vi "AddOption_Axes.vi"(0 "reference in":refnum<class "HTMLPlot.lvclass">, 2 "OptionsIn":string[](array[string]), 5 "error in (no error)":errorcluster) -> (14 "reference out":refnum<class "HTMLPlot.lvclass">, 16 "OptionsOut":string[](array[string]), 19 "error out":errorcluster)   [LabVIEW 2019, in "HTMLPlot.lvclass"]
uses:
  HTMLPlot.lvclass
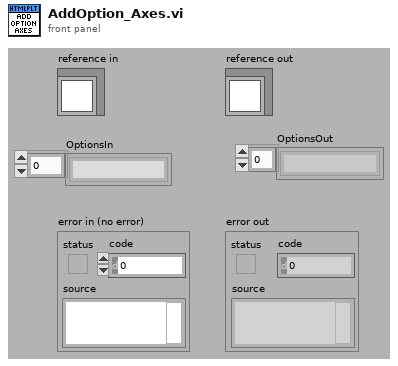
[diagram p1: front panel]
types:
  T1 = typedef "HTMLPlot.lvclass/ObjectAttributes.ctl" = cluster{"Attribute1":dbl, "GraphContainer":refnum<k7>, "ChartScriptFile":string, "UtilScriptFile(demoData)":string, "BaseHTML":string, "GenericProperties":cluster{"PlotType":T2, "PlotTitle":string, "XLabel":string, "YLabel":string, "ShowToolTip":bool}, "LegendProperties":cluster{"Show":bool, "Position":T3}, "BarPlot":cluster{"Dataset":dbl[][], "DatasetLabels":string[], "XLabels":string[], "PlotColours":u32[], "Stacked":bool}, "PiePlot":cluster{"Dataset":dbl[][], "DatasetLabels":string[], "PlotColours":u32[], "DoughnutStyle":bool, "PlotLabels":string[]}, "connection ID":refnum<k5>, "PortID":u64}
  T2 = typedef "HTMLPlot.lvclass/PlotType.ctl" = enum16{"bar", "line", "pie"}
  T3 = typedef "HTMLPlot.lvclass/LegendPosition.ctl" = enum16{"top", "right", "left", "bottom"}
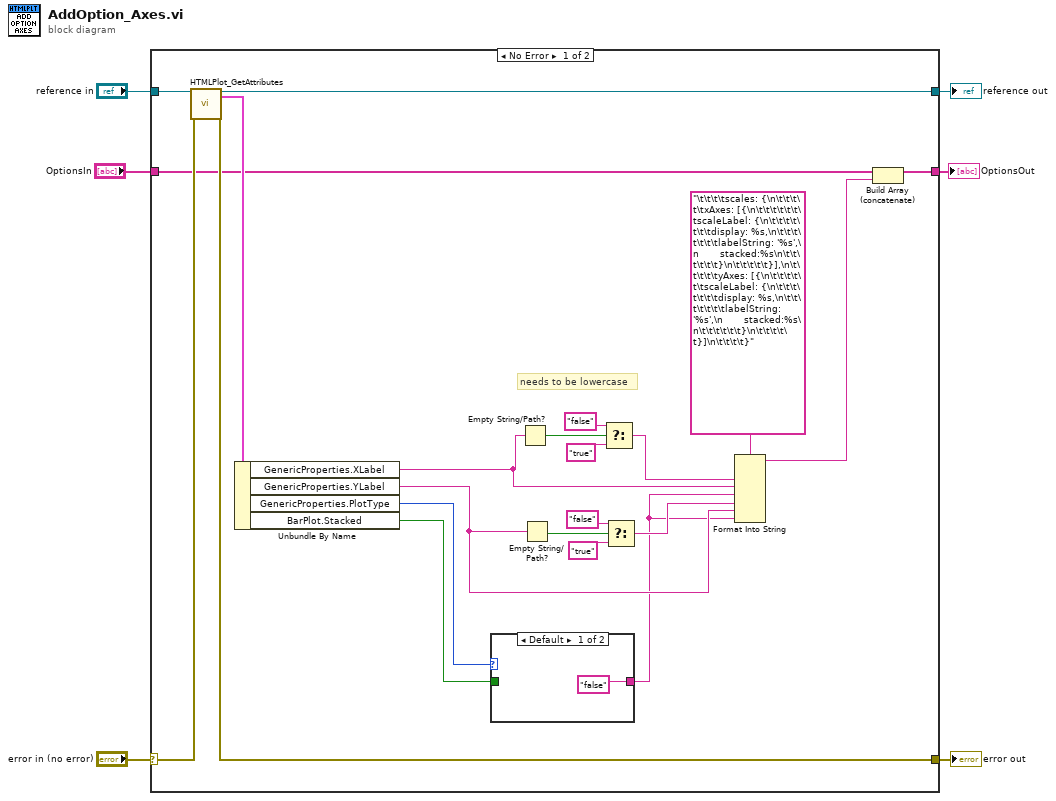
[diagram p0: block diagram]
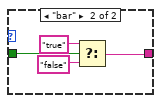
[diagram p2: hidden frame]
diagram:
  n1 = case shown="No Error" "error in (no error)" {
    selector: "error in (no error)" -> [w28 w36]
    tunnel: [w26 w36] -> w5
    tunnel: [w24 w35] -> w3
    tunnel: "reference in" -> [w25 w35]
    tunnel: "OptionsIn" -> [w23 w34]
    tunnel: [w22 w34] -> w1
    frame No Error {
      # "needs to be lowercase"
      n2 = call "HTMLPlot_GetAttributes.vi"("reference in"=w25, "error in (no error)"=w28) -> ("reference out"=w24:refnum<class "HTMLPlot.lvclass">, "Data"=w27:T1, "error out"=w26:errorcluster)  [unwired: 14 in, 1 out]
      n3 = Unbundle By Name(w27) -> ("GenericProperties.XLabel"=w12:string, "GenericProperties.YLabel"=w10:string, "GenericProperties.PlotType"=w9:T2, "BarPlot.Stacked"=w8:bool)
      n4 = case shown="Default" w9 {
        tunnel: w8 -> [_ w31]
        tunnel: ["false" w30] -> w7
        frame Default {
        }
        frame "bar" {
          n5 = Select(t="true", s=w31, f="false") -> (s? t:f=w30:string)
        }
      }
      n6 = Empty String/Path?(string/path=w12) -> (empty?=w16:bool)
      n7 = Empty String/Path?(string/path=w10) -> (empty?=w15:bool)
      n8 = Select(t="false", s=w16, f="true") -> (s? t:f=w17:string)
      n9 = Select(t="false", s=w15, f="true") -> (s? t:f=w11:string)
      n10 = Format Into String(format string="\t\t\t\tscales: {\n\t\t\t\t\txAxes: [{\n\t\t\t\t\t\t\tscaleLabel: {\n\t\t\t\t\t\t\tdisplay: %s,\n\t\t\t\t\t\t\tlabelString: '%s',\n       stacked:%s\n\t\t\t\t\t\t}\n\t\t\t\t\t}],\n\t\t\t\t\tyAxes: [{\n\t\t\t\t\t\tscaleLabel: {\n\t\t\t\t\t\t\tdisplay: %s,\n\t\t\t\t\t\t\tlabelString: '%s',\n       stacked:%s\n\t\t\t\t\t\t}\n\t\t\t\t\t}]\n\t\t\t\t}", w17, w12, w7, w11, w10, w7) -> (resulting string=w20:string)  [unwired: 2 in, 1 out]
      n11 = Build Array (concatenate)(w23, w20) -> (w22:string[])
    }
    frame Error {
    }
  }
  "error out" <- w5
  "reference out" <- w3
  "OptionsOut" <- w1
